vi "MSScript_SubVI_ArrayVarUpdValue.vi"(2 "new variable":ext[](array[numeric]), 3 "index arr":u32[](array[numeric]), 4 "@name":string) -> (0 "error":bool)   [LabVIEW 2018, in "MSScript.lvclass"]
uses:
  MSScript.lvclass
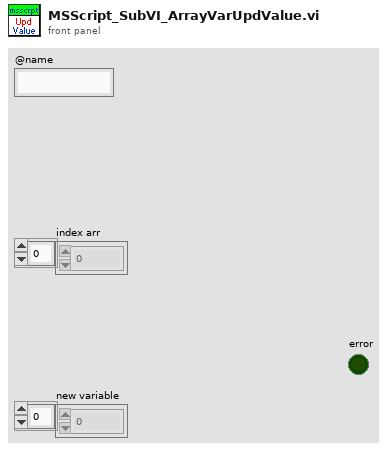
[diagram p1: front panel]
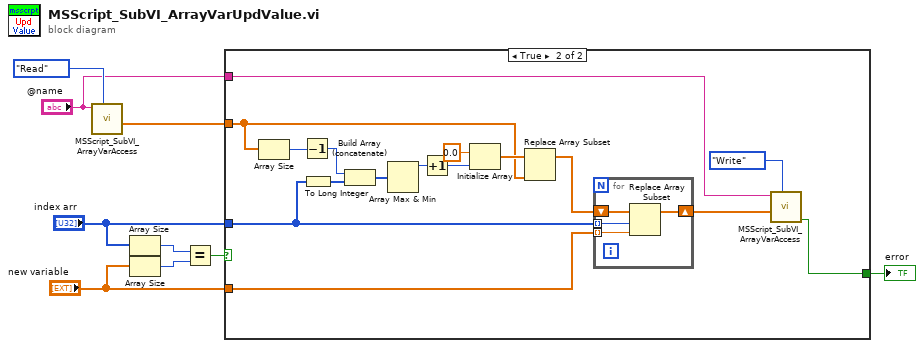
[diagram p0: block diagram]
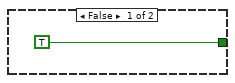
[diagram p2: hidden frame]
diagram:
  n1 = call "MSScript_SubVI_ArrayVarAccess.vi"("Function (Read)"=enum16{"Init", "Write", "Read"}."Read", "VarName"="@name") -> ("ArrayVariable out"=w8:ext[])  [unwired: 5 in, 2 out]
  n2 = Array Size(array="index arr") -> (size(s)=w7:i32)
  n3 = Array Size(array="new variable") -> (size(s)=w6:i32)
  n4 = Equal?(x=w7, y=w6) -> (x = y?=w4:bool)
  n5 = case shown="True" w4 {
    tunnel: w8 -> [_ w21]
    tunnel: "index arr" -> [_ w19]
    tunnel: "new variable" -> [_ w18]
    tunnel: [TRUE w13] -> w2
    tunnel: "@name" -> [_ w12]
    frame False {
    }
    frame True {
      n6 = Array Size(array=w21) -> (size(s)=w25:i32)
      n7 = Decrement(x=w25) -> (x-1=w11:i32)
      n8 = To Long Integer(number=w19) -> (32bit integer=w23:i32[])
      n9 = Build Array (concatenate)(w11, w23) -> (w24:i32[])
      n10 = Array Max & Min(array=w24) -> (max value=w17:i32)  [unwired: 3 out]
      n11 = Increment(x=w17) -> (x+1=w16:i32)
      n12 = Initialize Array(0.0 ("element"), w16) -> (w22:dbl[])
      n13 = Replace Array Subset(array=w22, new element=w21) -> (w20:dbl[])  [unwired: 1 in]
      n14 = for {
        tunnel: w19 -> [w29] mode=indexing
        tunnel: w18 -> [w28] mode=indexing
        shift-right: [w27] -> w14
        shift-left: w20 -> [w30]
        n15 = Replace Array Subset(array=w30, new element=w28, index=w29) -> (w27:dbl[])
      }
      n16 = call "MSScript_SubVI_ArrayVarAccess.vi"("Function (Read)"=enum16{"Init", "Write", "Read"}."Write", "ArrayVariable in"=w14, "VarName"=w12) -> ("Value Error?"=w13:bool)  [unwired: 4 in, 2 out]
    }
  }
  "error" <- w2
